vi "Difference.vi"(10 "Angle":dbl, 11 "Gyro":dbl) -> (3 "Difference":dbl)   [LabVIEW 2020]
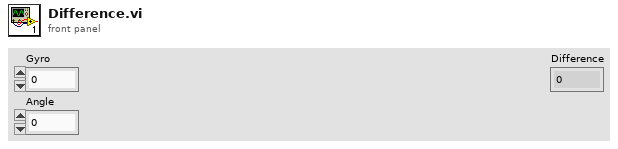
[diagram p1: front panel]
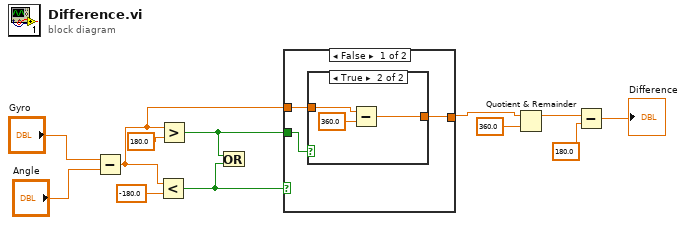
[diagram p0: block diagram]
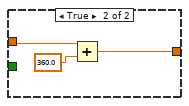
[diagram p3: hidden frame]
diagram:
  n1 = Subtract(x="Gyro", y="Angle") -> (x-y=w6:dbl)
  n2 = Less?(x=w6, y=-180.0) -> (x < y?=w8:bool)
  n3 = Greater?(x=w6, y=180.0) -> (0:w7:bool)
  n4 = Or(x=w7, y=w8) -> ()  [unwired: 1 out]
  n5 = case shown="False" w8 {
    tunnel: w7 -> [w15 _]
    tunnel: w6 -> [w14 w22]
    tunnel: [w13 w20] -> w1
    frame False {
      n6 = case shown="True" w15 {
        tunnel: w14 -> [w16 w18]
        tunnel: [w16 w17] -> w13
        frame False {
        }
        frame True {
          n7 = Subtract(x=w18, y=360.0) -> (x-y=w17:dbl)
        }
      }
    }
    frame True {
      n8 = Add(x=w22, y=360.0) -> (x+y=w20:dbl)
    }
  }
  n9 = Quotient & Remainder(x=w1, y=360.0) -> (x-y*floor(x/y)=w2:dbl)  [unwired: 1 out]
  n10 = Subtract(x=w2, y=180.0) -> (x-y=→"Difference":dbl)
